vi "Initialize Instrument.vi"(8 "error in (no error)":errorcluster, 10 "Reset":bool, 11 "Keithley 648x in":refnum<class "Keithley 648x.lvclass">) -> (0 "error out":errorcluster, 3 "Keithley 648x out":refnum<class "Keithley 648x.lvclass">)   [LabVIEW 2020, in "Keithley 648x.lvclass"]
uses:
  Keithley 648x.lvclass
  C:/Sandbox/Git_Sandbox/WiSpry Test Framework source code (LV20)/WiSpry Test Framework/Instruments/Instrument.lvclass
  C:/Sandbox/Git_Sandbox/WiSpry Test Framework source code (LV20)/WiSpry Test Framework/Instruments/Power Supply/Power Supply.lvclass
  Instrument.lvclass/Instrument.ctl
  Power Supply.lvclass/Power Supply.ctl
  Instrument.lvclass
  Power Supply.lvclass
  <instrlib>/Keithley 648X Series/Keithley 648X Series.lvlib
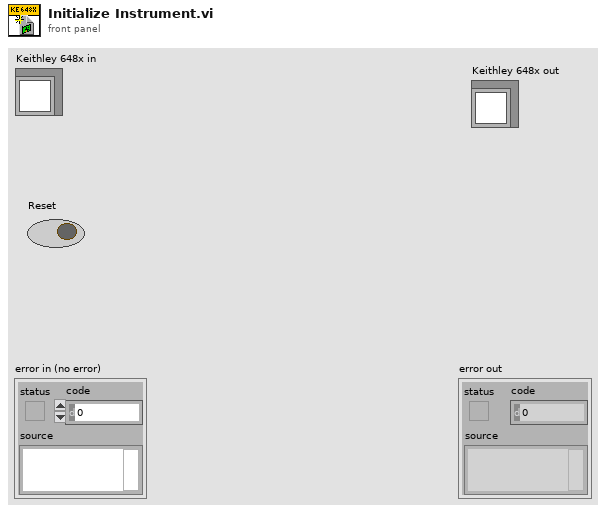
[diagram p1: front panel]
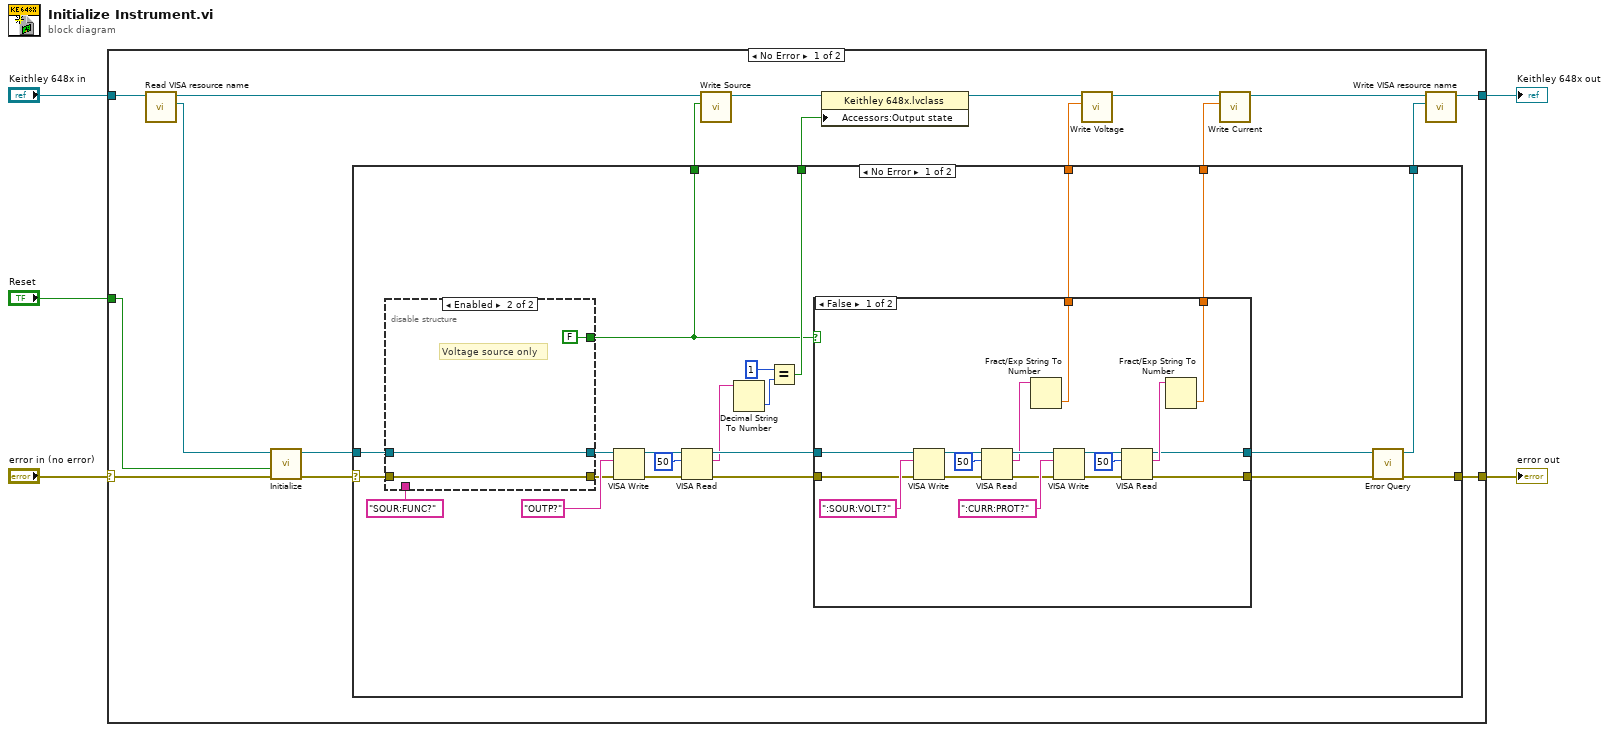
[diagram p0: block diagram]
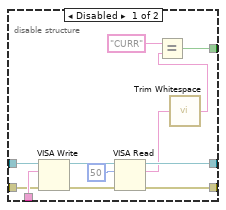
[diagram p2: hidden frame]
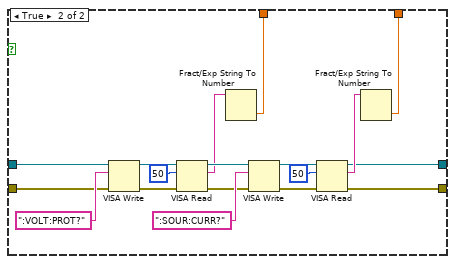
[diagram p3: hidden frame]
diagram:
  n1 = case shown="No Error" "error in (no error)" {
    selector: "error in (no error)" -> [w8 w100]
    tunnel: [w22 w100] -> w2
    tunnel: [w23 w99] -> w1
    tunnel: "Reset" -> [w7 _]
    tunnel: "Keithley 648x in" -> [w20 w99]
    frame No Error {
      n2 = call "Read VISA resource name.vi"("Instrument in"=w20) -> ("VISA resource name"=w9:refnum<visa-resource-name>, "Instrument out"=w14:refnum<class "Keithley 648x.lvclass">)  [unwired: 9 in]
      n3 = call <instrlib>:"Initialize.vi"("error in (no error)"=w8, "Reset (True)"=w7, "VISA resource name"=w9) -> ("error out"=w11:errorcluster, "VISA resource name out"=w10:refnum<visa-resource-name>)  [unwired: 7 in]
      n4 = case shown="No Error" w11 {
        selector: w11 -> [w28 w98]
        tunnel: [w24 w98] -> w22
        tunnel: [w25 w97] -> w21
        tunnel: [w33 _] -> w17
        tunnel: [w32 _] -> w16
        tunnel: [w31 _] -> w6
        tunnel: [w30 _] -> w12
        tunnel: w10 -> [w29 w97]
        frame No Error {
          n5 = disable-structure shown="Enabled" {
            disable-tunnel: "SOUR:FUNC?" ("write buffer") -> [w57 _]
            disable-tunnel: [w53 w60] -> w35
            disable-tunnel: [w52 w59] -> w34
            disable-tunnel: [w50 FALSE] -> w30
            disable-tunnel: w29 -> [w47 w59]
            disable-tunnel: w28 -> [w46 w60]
            frame Disabled {
              n6 = VISA Write(VISA resource name=w47, write buffer=w57, error in (no error)=w46) -> (VISA resource name out=w55:refnum<visa-resource-name>, error out=w54:errorcluster)  [unwired: 1 out]
              n7 = VISA Read(VISA resource name=w55, byte count=u32 50, error in (no error)=w54) -> (VISA resource name out=w52:refnum<visa-resource-name>, read buffer=w49:string, error out=w53:errorcluster)  [unwired: 1 out]
              n8 = call <vilib>:"Trim Whitespace.vi"("string"=w49) -> ("trimmed string"=w48:string)  [unwired: 1 in]
              n9 = Equal?(x="CURR", y=w48) -> (x = y?=w50:bool)
            }
            frame Enabled {
              # "Voltage source only"
            }
          }
          n10 = VISA Write(VISA resource name=w34, write buffer="OUTP?", error in (no error)=w35) -> (VISA resource name out=w45:refnum<visa-resource-name>, error out=w44:errorcluster)  [unwired: 1 out]
          n11 = VISA Read(VISA resource name=w45, byte count=u32 50, error in (no error)=w44) -> (VISA resource name out=w41:refnum<visa-resource-name>, read buffer=w39:string, error out=w40:errorcluster)  [unwired: 1 out]
          n12 = Decimal String To Number(string=w39) -> (number=w38:i32)  [unwired: 2 in, 1 out]
          n13 = Equal?(x=1, y=w38) -> (x = y?=w31:bool)
          n14 = case shown="False" w30 {
            tunnel: w41 -> [w70 w88]
            tunnel: w40 -> [w69 w87]
            tunnel: [w64 w82] -> w27
            tunnel: [w63 w81] -> w26
            tunnel: [w62 w80] -> w33
            tunnel: [w61 w79] -> w32
            frame False {
              n15 = VISA Write(VISA resource name=w70, write buffer=":SOUR:VOLT?", error in (no error)=w69) -> (VISA resource name out=w75:refnum<visa-resource-name>, error out=w76:errorcluster)  [unwired: 1 out]
              n16 = VISA Read(VISA resource name=w75, byte count=u32 50, error in (no error)=w76) -> (VISA resource name out=w68:refnum<visa-resource-name>, read buffer=w65:string, error out=w67:errorcluster)  [unwired: 1 out]
              n17 = Fract/Exp String To Number(string=w65) -> (number=w62:dbl)  [unwired: 3 in, 1 out]
              n18 = VISA Write(VISA resource name=w68, write buffer=":CURR:PROT?", error in (no error)=w67) -> (VISA resource name out=w74:refnum<visa-resource-name>, error out=w73:errorcluster)  [unwired: 1 out]
              n19 = VISA Read(VISA resource name=w74, byte count=u32 50, error in (no error)=w73) -> (VISA resource name out=w63:refnum<visa-resource-name>, read buffer=w66:string, error out=w64:errorcluster)  [unwired: 1 out]
              n20 = Fract/Exp String To Number(string=w66) -> (number=w61:dbl)  [unwired: 3 in, 1 out]
            }
            frame True {
              n21 = VISA Write(VISA resource name=w88, write buffer=":VOLT:PROT?", error in (no error)=w87) -> (VISA resource name out=w93:refnum<visa-resource-name>, error out=w94:errorcluster)  [unwired: 1 out]
              n22 = VISA Read(VISA resource name=w93, byte count=u32 50, error in (no error)=w94) -> (VISA resource name out=w86:refnum<visa-resource-name>, read buffer=w83:string, error out=w85:errorcluster)  [unwired: 1 out]
              n23 = Fract/Exp String To Number(string=w83) -> (number=w80:dbl)  [unwired: 3 in, 1 out]
              n24 = VISA Write(VISA resource name=w86, write buffer=":SOUR:CURR?", error in (no error)=w85) -> (VISA resource name out=w92:refnum<visa-resource-name>, error out=w91:errorcluster)  [unwired: 1 out]
              n25 = VISA Read(VISA resource name=w92, byte count=u32 50, error in (no error)=w91) -> (VISA resource name out=w81:refnum<visa-resource-name>, read buffer=w84:string, error out=w82:errorcluster)  [unwired: 1 out]
              n26 = Fract/Exp String To Number(string=w84) -> (number=w79:dbl)  [unwired: 3 in, 1 out]
            }
          }
          n27 = call <instrlib>:"Error Query.vi"("error in (no error)"=w27, "VISA resource name"=w26) -> ("error out"=w24:errorcluster, "VISA resource name out"=w25:refnum<visa-resource-name>)  [unwired: 6 in, 2 out]
        }
        frame Error {
        }
      }
      n28 = call-dynamic "Write Source.vi"("Source"=w12, "Power Supply in"=w14) -> ("Power Supply out"=w15:refnum<class "Keithley 648x.lvclass">)  [unwired: 9 in]
      n29 = property class="Keithley 648x.lvclass"(reference=w15, "Accessors:Output state"=w6) -> (reference out=w19:refnum<class "Keithley 648x.lvclass">)  [unwired: 1 in, 1 out]
      n30 = call "Write Voltage.vi"("Voltage"=w17, "Power Supply in"=w19) -> ("Power Supply out"=w18:refnum<class "Keithley 648x.lvclass">)  [unwired: 9 in]
      n31 = call "Write Current.vi"("Current"=w16, "Power Supply in"=w18) -> ("Power Supply out"=w13:refnum<class "Keithley 648x.lvclass">)  [unwired: 9 in]
      n32 = call "Write VISA resource name.vi"("VISA resource name"=w21, "Instrument in"=w13) -> ("Instrument out"=w23:refnum<class "Keithley 648x.lvclass">)  [unwired: 9 in]
    }
    frame Error {
    }
  }
  "error out" <- w2
  "Keithley 648x out" <- w1
